vi "zmq atomic counter set.vi"(8 "error in (no error)":errorcluster, 10 "value_":i32, 11 "counter_":u32) -> (0 "error out":errorcluster, 3 "counter_ out":u32)   [LabVIEW 2025, in "libzmq-v143-mt-4_3_6.lvlib"]
doc: "ZMQ_EXPORT void zmq_atomic_counter_set (void *counter_, int value_);"
uses:
  libzmq-v143-mt-4_3_6.lvlib
  LV/LibZMQ/libzmq/lv_x86/bin/Release/libzmq-v143-mt-4_3_6.dll
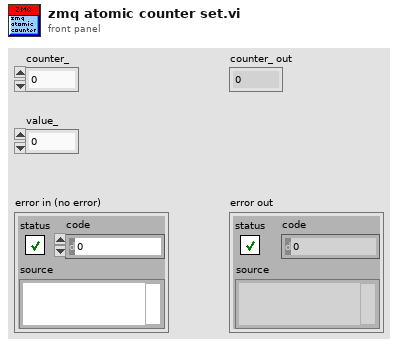
[diagram p1: front panel]
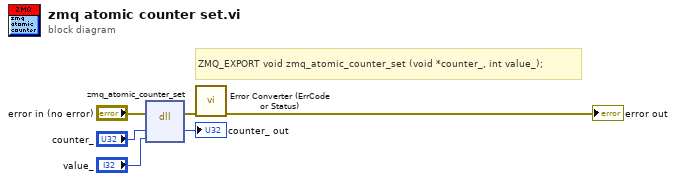
[diagram p0: block diagram]
diagram:
  # "ZMQ_EXPORT void zmq_atomic_counter_set (void *counter_, int value_);"
  n1 = dll-call lib="C:/LV/LibZMQ/libzmq/lv_x86/bin/Release/libzmq-v143-mt-4_3_6.*" fn="zmq_atomic_counter_set"(error in="error in (no error)", "counter_"="counter_", "value_"="value_") -> (error out=w2:errorcluster, "counter_"=→"counter_ out":u32)  [unwired: 4 in, 1 out]
  n2 = call "Error Converter (ErrCode or Status).vi"("error in (no error)"=w2) -> ("error out"=→"error out":errorcluster)  [unwired: 10 in]
